vi "Add spaces.vi"(9 "spaces no":i32, 11 "input string":string) -> (3 "result string":string)   [LabVIEW 2019, in "infolib.lvlib"]
doc: "Add desired number of spaces at the beginning of every line in input string."
uses:
  infolib.lvlib
panel:
  # "test string:"
  # "aa\\r\\nbb\\r\\ncc"
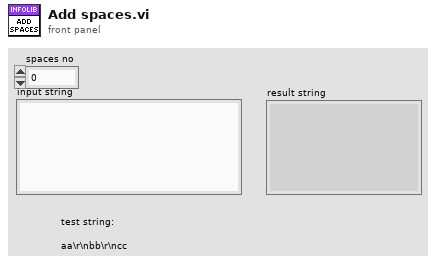
[diagram p1: front panel]
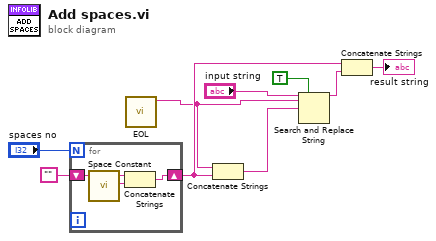
[diagram p0: block diagram]
diagram:
  n1 = for {
    N: "spaces no" -> [_]
    shift-right: [w10] -> w4
    shift-left: "" -> [w11]
    n2 = call <vilib>:"Space Constant.vi"() -> ("String"=w12:string)
    n3 = Concatenate Strings(w11, w12) -> (w10:string)
  }
  n4 = call "EOL.vi"() -> ("eol"=w1:string)  [unwired: 11 in]
  n5 = Concatenate Strings(w1, w4) -> (w5:string)
  n6 = Search and Replace String(replace all?=TRUE ("replace all? (F)"), input string="input string", search string=w1, replace string=w5) -> (result string=w3:string)  [unwired: 4 in, 3 out]
  n7 = Concatenate Strings(w4, w3) -> (→"result string":string)
